vi "Unreserve Resource.vi"(8 "error in (no error)":errorcluster, 9 "Name in Bitfile":string, 10 "Server Ref in":T1 format="%.0x", 11 "Item Ref in":T1 format="%.0x") -> (0 "error out":errorcluster, 3 "Item Ref out":T1 format="%.0x")   [LabVIEW 2016, in "FPGA RM System Definition API.lvlib"]
uses:
  System Definition/FPGA RM System Definition API.lvlib
  <vilib>/NI Veristand/Custom Device API/Custom Device Item Ref.ctl
  <vilib>/NI VeriStand/Custom Device API/Custom Device API.lvlib
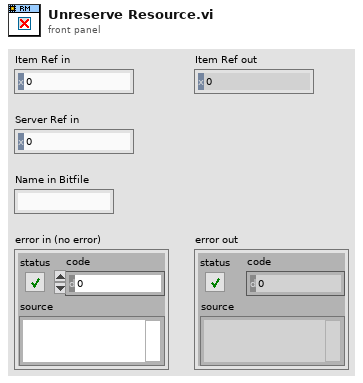
[diagram p1: front panel]
types:
  T1 = typedef "Custom Device API.lvlib/Custom Device Item Ref.ctl" = u64
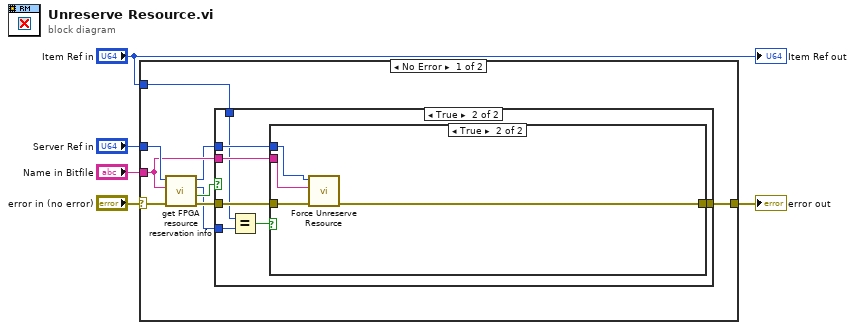
[diagram p0: block diagram]
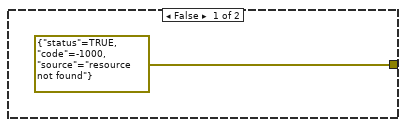
[diagram p2: hidden frame]
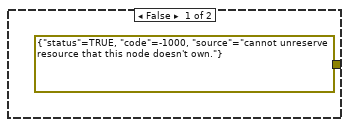
[diagram p3: hidden frame]
diagram:
  n1 = case shown="No Error" "error in (no error)" {
    selector: "error in (no error)" -> [w11 w28]
    tunnel: [w14 w28] -> w4
    tunnel: "Item Ref in" -> [w7 _]
    tunnel: "Server Ref in" -> [w13 _]
    tunnel: "Name in Bitfile" -> [w12 _]
    frame No Error {
      n2 = call "get FPGA resource reservation info.vi"("error in (no error)"=w11, "Name in Bitfile"=w12, "Item Ref in"=w13) -> ("error out"=w10:errorcluster, "found?"=w9:bool, "Reserver Node Ref"=w8:T1, "Item Ref out"=w6:T1)  [unwired: 3 in, 2 out]
      n3 = case shown="True" w9 {
        tunnel: [errorcluster {"status"=TRUE, "code"=-1000, "source"="resource not found"} ("error out") w22] -> w14
        tunnel: w6 -> [_ w21]
        tunnel: w12 -> [_ w20]
        tunnel: w10 -> [_ w19]
        tunnel: w8 -> [_ w17]
        tunnel: w7 -> [_ w16]
        frame False {
        }
        frame True {
          n4 = Equal?(x=w16, y=w17) -> (x = y?=w18:bool)
          n5 = case shown="True" w18 {
            tunnel: [errorcluster {"status"=TRUE, "code"=-1000, "source"="cannot unreserve resource that this node doesn't own."} ("error out") w27] -> w22
            tunnel: w21 -> [_ w26]
            tunnel: w20 -> [_ w25]
            tunnel: w19 -> [_ w24]
            frame False {
            }
            frame True {
              n6 = call "Force Unreserve Resource.vi"("error in (no error)"=w24, "Name in bitfile"=w25, "Item Ref in"=w26) -> ("error out"=w27:errorcluster)  [unwired: 7 in, 1 out]
            }
          }
        }
      }
    }
    frame Error {
    }
  }
  "error out" <- w4
  "Item Ref out" <- "Item Ref in"
